vi "PID_VI_edits_feb3.vi"(5 "Integral allowed?":bool, 7 "PID gains":T1={"proportional gain (Kc)"=1.0, "integral time (Ti, min)"=0.01, "derivative time (Td, min)"=0.0} {"derivative time (Td, min)" format="%.3f"; "integral time (Ti, min)" format="%.3f"; "proportional gain (Kc)" format="%.3f"}, 8 "dt (s)":dbl=-1.0 format="%.3f", 9 "reinitialize? (F)":bool, 10 "process variable":dbl format="%.2f", 11 "setpoint":dbl format="%.2f") -> (0 "dt out (s)":dbl format="%.3f", 1 "output":dbl format="%.2f", 2 "Integrated error":dbl)   [LabVIEW 2019]
uses:
  Global 9.vi
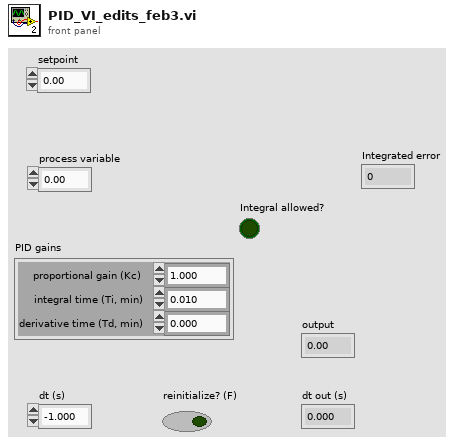
[diagram p1: front panel]
types:
  T1 = cluster{"proportional gain (Kc)":dbl, "integral time (Ti, min)":dbl, "derivative time (Td, min)":dbl}
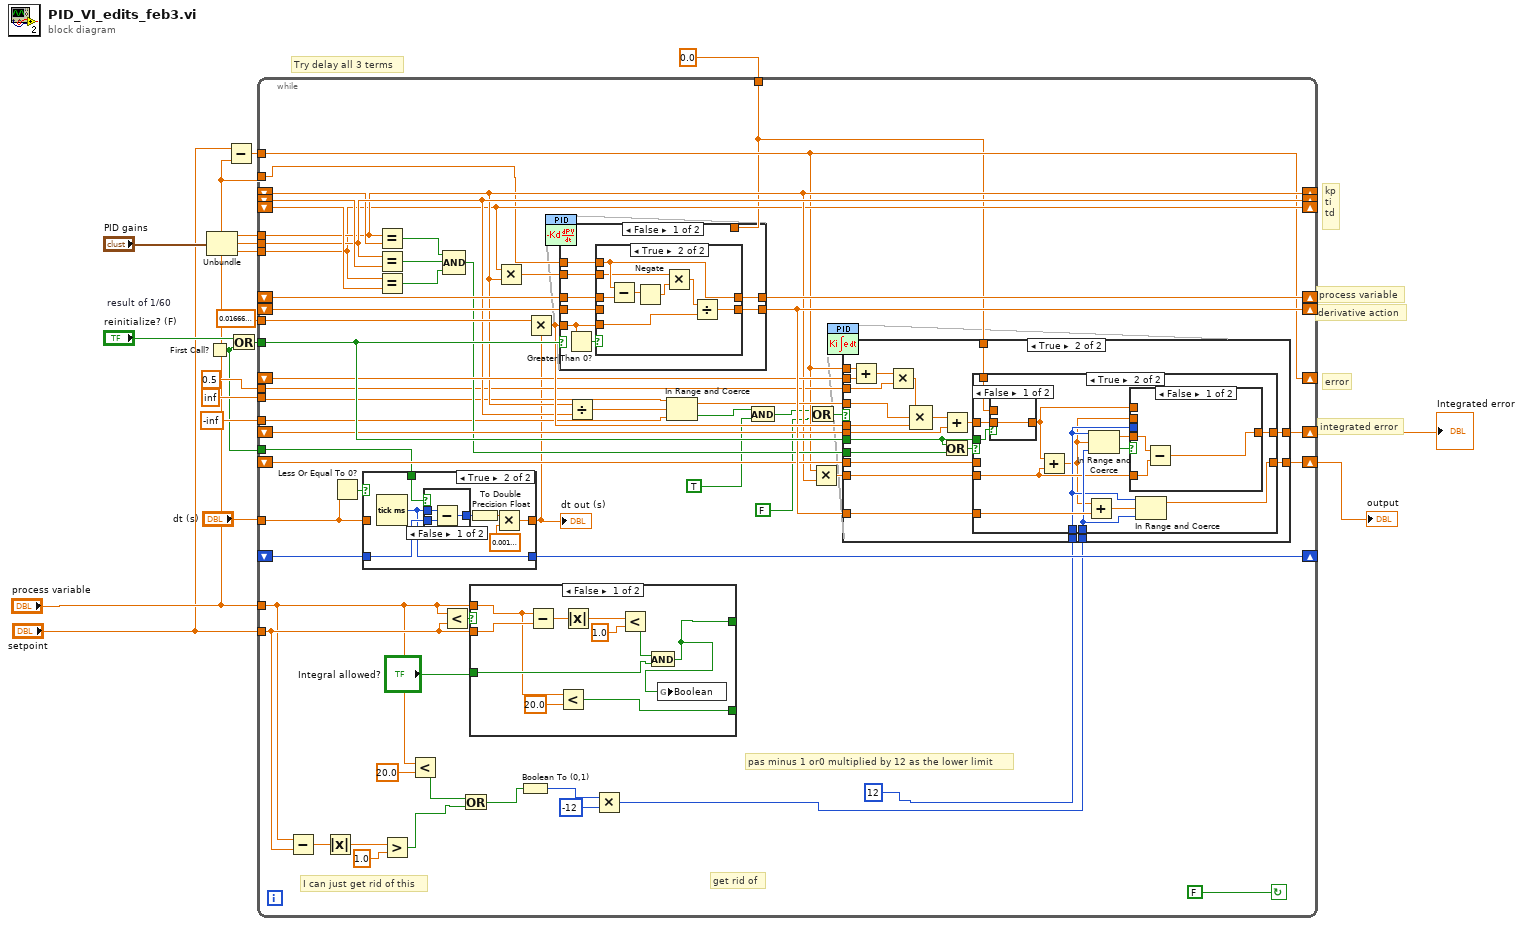
[diagram p0: block diagram]
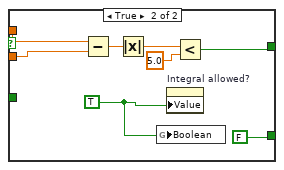
[diagram p2: hidden frame]
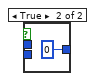
[diagram p4: hidden frame]
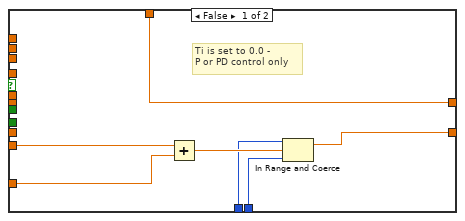
[diagram p5: hidden frame]
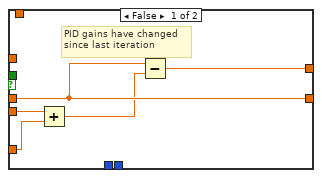
[diagram p6: hidden frame]
diagram:
  w14 = 0.016666666666666666  # result of 1/60
  # "Try delay all 3 terms"
  # "derivative action"
  # "process variable"
  # "kp\nti\ntd"
  # "error"
  # "integrated error"
  n1 = First Call?() -> (First Call?: T/F=w5:bool)
  n2 = Unbundle("PID gains") -> ("proportional gain (Kc)"=w17:dbl, "integral time (Ti, min)"=w16:dbl, "derivative time (Td, min)"=w15:dbl)
  n3 = Subtract(x="setpoint", y="process variable") -> (x-y=w7:dbl)
  n4 = Or(x="reinitialize? (F)", y=w5) -> (x .or. y?=w18:bool)
  n5 = while {
    tunnel: w18 -> [w77]
    shift-left: _ -> [w43]
    shift-right: [w44] -> _
    shift-right: [w53] -> _
    shift-left: _ -> [w54]
    shift-right: [w55] -> _
    shift-left: _ -> [w74]
    shift-right: [w48] -> _
    shift-left: _ -> [w75]
    tunnel: w17 -> [w53]
    tunnel: w16 -> [w55]
    tunnel: w15 -> [w48]
    tunnel: "dt (s)" -> [w42]
    tunnel: "process variable" -> [w28]
    shift-right: [w70] -> _
    shift-left: _ -> [w69]
    shift-right: [w68] -> _
    shift-left: _ -> [w61]
    shift-right: [w67] -> w4
    shift-left: _ -> [w66]
    shift-right: [w47] -> _
    shift-left: _ -> [w65]
    shift-right: [w64] -> w2
    shift-left: _ -> [w63]
    tunnel: w14 -> [w58]
    tunnel: 0.5 ("y") -> [w52]
    tunnel: inf ("upper limit") -> [w50]
    tunnel: -inf ("lower limit") -> [w51]
    tunnel: w7 -> [w47]
    tunnel: 0.0 -> [w46]
    tunnel: w5 -> [w40]
    tunnel: "process variable" -> [w32]
    tunnel: "setpoint" -> [w34]
    stop <- FALSE continue-if-true
    # "get rid of"
    # "I can just get rid of this"
    # "pas minus 1 or0 multiplied by 12 as the lower limit"
    n6 = Subtract(x=w32, y=w34) -> (x-y=w37:dbl)
    n7 = Absolute Value(x=w37) -> (abs(x)=w36:dbl)
    n8 = Less Or Equal To 0?(x=w42) -> (x <= 0?=w41:bool)
    n9 = case shown="True" w41 {
      tunnel: [w97 w101] -> w45
      tunnel: w43 -> [w96 w100]
      tunnel: [w96 w99] -> w44
      tunnel: w42 -> [w97 _]
      tunnel: w40 -> [_ w98]
      frame False {
      }
      frame True {
        n10 = Tick Count (ms)() -> (millisecond timer value=w99:u32)
        n11 = case shown="False" w98 {
          tunnel: [w107 u32 0] -> w103
          tunnel: w100 -> [w106 _]
          tunnel: w99 -> [w105 _]
          frame False {
            n12 = Subtract(x=w105, y=w106) -> (x-y=w107:u32)
          }
          frame True {
          }
        }
        n13 = To Double Precision Float(number=w103) -> (double precision float=w102:dbl)
        n14 = Multiply(x=w102, y=0.0010000000474974513) -> (x*y=w101:dbl)
      }
    }
    "dt out (s)" <- w45
    n15 = Equal?(x=w53, y=w54) -> (x = y?=w72:bool)
    n16 = Equal?(x=w55, y=w74) -> (x = y?=w71:bool)
    n17 = Equal?(x=w48, y=w75) -> (x = y?=w73:bool)
    n18 = Greater?(x=w36, y=1.0) -> (0:w19:bool)
    n19 = Less?(x=w32, y=20.0) -> (x < y?=w33:bool)
    n20 = Less?(x=w32, y=w34) -> (x < y?=w38:bool)
    n21 = Compound Arithmetic op=AND(w72, w71, w73) -> (w56:bool)
    n22 = Or(x=w33, y=w19) -> (x .or. y?=w24:bool)
    n23 = case shown="False" w38 {
      tunnel: [w81 w94] -> _
      tunnel: w32 -> [w80 w93]
      tunnel: w34 -> [w84 w92]
      tunnel: "Integral allowed?" -> [w82 _]
      tunnel: [w78 FALSE] -> _
      frame False {
        n24 = Subtract(x=w80, y=w84) -> (x-y=w87:dbl)
        n25 = Less?(x=w80, y=20.0) -> (x < y?=w78:bool)
        n26 = Absolute Value(x=w87) -> (abs(x)=w86:dbl)
        n27 = Less?(x=w86, y=1.0) -> (x < y?=w83:bool)
        n28 = And(x=w83, y=w82) -> (x .and. y?=w81:bool)
        n29 = global write "Global 9.vi" "Boolean"(w81) -> ()
      }
      frame True {
        w89 = TRUE
        n30 = Subtract(x=w93, y=w92) -> (x-y=w91:dbl)
        n31 = Absolute Value(x=w91) -> (abs(x)=w90:dbl)
        n32 = global write "Global 9.vi" "Boolean"(w89) -> ()
        n33 = property on="Integral allowed?" class="Bool (strict)"("Value"=w89) -> ()  [unwired: 2 in, 2 out]
        n34 = Less?(x=w90, y=5.0) -> (x < y?=w94:bool)
      }
    }
    n35 = Multiply(x=w48, y=w53) -> (x*y=w60:dbl)
    n36 = Boolean To (0,1)(Boolean=w24) -> (0, 1=w22:i16)
    n37 = Multiply(x=w58, y=w45) -> (x*y=w76:dbl)
    n38 = case shown="False" w77 {
      tunnel: w69 -> [w169 _]
      tunnel: w60 -> [w166 _]
      tunnel: w28 -> [w168 w181]
      tunnel: [w165 w181] -> w70
      tunnel: [w167 w180] -> w68
      tunnel: w61 -> [w163 _]
      tunnel: w76 -> [w162 _]
      tunnel: w46 -> [_ w180]
      frame False {
        n39 = Greater Than 0?(x=w162) -> (x > 0?=w164:bool)
        n40 = case shown="True" w164 {
          tunnel: w169 -> [w171 w177]
          tunnel: w162 -> [_ w176]
          tunnel: w168 -> [_ w174]
          tunnel: [w170 w175] -> w167
          tunnel: w166 -> [_ w172]
          tunnel: [w171 w174] -> w165
          tunnel: w163 -> [w170 _]
          frame False {
            # "dt = 0 min"
          }
          frame True {
            n41 = Subtract(x=w174, y=w177) -> (x-y=w179:dbl)
            n42 = Negate(x=w179) -> (-x=w173:dbl)
            n43 = Multiply(x=w172, y=w173) -> (x*y=w178:dbl)
            n44 = Divide(x=w178, y=w176) -> (x/y=w175:dbl)
          }
        }
      }
      frame True {
      }
    }
    n45 = Divide(x=w53, y=w55) -> (x/y=w59:dbl)
    n46 = Multiply(x=w22, y=i16 -12) -> (x*y=w20:i16)
    n47 = In Range and Coerce(upper limit=w50, x=w59, lower limit=w51) -> (coerced(x)=w62:dbl, In Range?=w39:bool)
    n48 = And(x=w39, y=TRUE) -> (x .and. y?=w30:bool)
    n49 = Or(x=w30, y=FALSE) -> (x .or. y?=w29:bool)
    n50 = Multiply(x=w47, y=w53) -> (x*y=w57:dbl)
    n51 = case shown="True" w29 {
      tunnel: w47 -> [_ w135]
      tunnel: w65 -> [_ w136]
      tunnel: w63 -> [_ w131]
      tunnel: [w109 w126] -> w64
      tunnel: w62 -> [_ w124]
      tunnel: w57 -> [w114 w129]
      tunnel: [w115 w125] -> w67
      tunnel: w66 -> [_ w127]
      tunnel: w68 -> [w113 w123]
      tunnel: w77 -> [_ w122]
      tunnel: w56 -> [_ w121]
      tunnel: w76 -> [_ w120]
      tunnel: 12 -> [w111 w118]
      tunnel: w20 -> [w110 w119]
      tunnel: w52 -> [_ w117]
      tunnel: w46 -> [w109 w116]
      frame False {
        # "Ti is set to 0.0 -\nP or PD control only"
        n52 = Add(x=w114, y=w113) -> (x+y=w112:dbl)
        n53 = In Range and Coerce(upper limit=w111, x=w112, lower limit=w110) -> (coerced(x)=w115:dbl)  [unwired: 1 out]
      }
      frame True {
        n54 = Add(x=w135, y=w136) -> (x+y=w134:dbl)
        n55 = Multiply(x=w134, y=w117) -> (x*y=w133:dbl)
        n56 = Compound Arithmetic op=MULTIPLY(w133, w124, w120) -> (w132:dbl)
        n57 = Add(x=w132, y=w131) -> (x+y=w130:dbl)
        n58 = Or(x=w122, y=w121) -> (x .or. y?=w128:bool)
        n59 = case shown="True" w128 {
          tunnel: w130 -> [_ w149]
          tunnel: w129 -> [w139 w144]
          tunnel: w127 -> [w141 _]
          tunnel: w122 -> [_ w151]
          tunnel: [w140 w146] -> w126
          tunnel: [w141 w154] -> w125
          tunnel: w123 -> [w138 w153]
          tunnel: w119 -> [_ w152]
          tunnel: w118 -> [_ w143]
          tunnel: w116 -> [_ w150]
          frame False {
            # "PID gains have changed\nsince last iteration"
            n60 = Add(x=w139, y=w138) -> (x+y=w137:dbl)
            n61 = Subtract(x=w141, y=w137) -> (x-y=w140:dbl)
          }
          frame True {
            n62 = case shown="False" w151 {
              tunnel: w150 -> [_ w161]
              tunnel: [w160 w161] -> w148
              tunnel: w149 -> [w160 _]
              frame False {
              }
              frame True {
              }
            }
            n63 = Add(x=w148, y=w144) -> (x+y=w142:dbl)
            n64 = Add(x=w142, y=w153) -> (x+y=w155:dbl)
            n65 = In Range and Coerce(upper limit=w143, x=w142, lower limit=w152) -> (coerced(x)=w145:dbl, In Range?=w147:bool)
            n66 = case shown="False" w147 {
              tunnel: w148 -> [_ w159]
              tunnel: [w156 w159] -> w146
              tunnel: w145 -> [w158 _]
              tunnel: w144 -> [w157 _]
              tunnel: w143 -> [_ _]
              tunnel: w142 -> [_ _]
              frame False {
                n67 = Subtract(x=w158, y=w157) -> (x-y=w156:dbl)
              }
              frame True {
              }
            }
            n68 = In Range and Coerce(upper limit=w143, x=w155, lower limit=w152) -> (coerced(x)=w154:dbl)  [unwired: 1 out]
          }
        }
      }
    }
  }
  "output" <- w4
  "Integrated error" <- w2
